vi "InitQueues.vi"(8 "error in (no error)":errorcluster) -> (0 "error out":errorcluster, 3 "Application Data":T1)   [LabVIEW 2019]
uses:
  Typedefs/#cluster_ApplicationData.ctl
  Typedefs/Acquisition Thread/#cluster_AcqQueueData.ctl
  Typedefs/Acquisition Thread/#enum_AcquisitionTask.ctl
  Typedefs/Saving Thread/#cluster_SavingQueueData.ctl
  Typedefs/Saving Thread/#enum_SavingTask.ctl
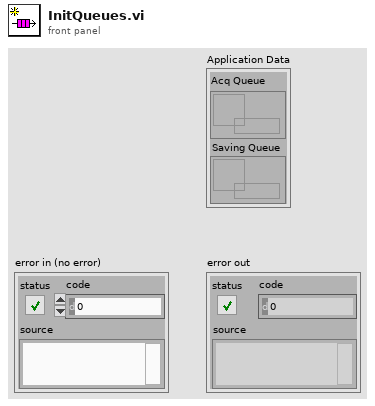
[diagram p1: front panel]
types:
  T1 = typedef "#cluster_ApplicationData.ctl" = cluster{"Acq Queue":refnum<queue>, "Saving Queue":refnum<queue>}
  T2 = typedef "#cluster_SavingQueueData.ctl" = cluster{"Task":T3, "Data":variant}
  T3 = typedef "#enum_SavingTask.ctl" = enum16{"Set directory", "Save", "Stop", "Close"}
  T4 = typedef "#cluster_AcqQueueData.ctl" = cluster{"Task":T5, "Data":variant}
  T5 = typedef "#enum_AcquisitionTask.ctl" = enum16{"Init", "Start", "Finish", "Close"}
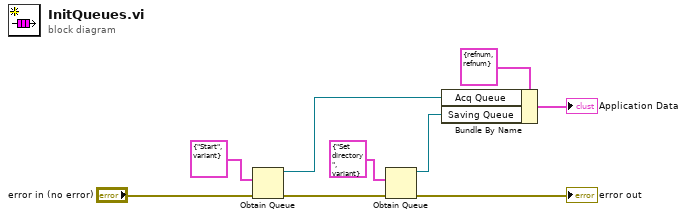
[diagram p0: block diagram]
diagram:
  n1 = Obtain Queue(element data type=T4 {"Task"=enum."Start", "Data"=variant} ("Acq Data"), error in (no error)="error in (no error)") -> (queue out=w5:refnum<queue>, error out=w8:errorcluster)  [unwired: 3 in, 1 out]
  n2 = Obtain Queue(element data type=T2 {"Task"=enum."Set directory", "Data"=variant} ("Saving Data"), error in (no error)=w8) -> (queue out=w4:refnum<queue>, error out=→"error out":errorcluster)  [unwired: 3 in, 1 out]
  n3 = Bundle By Name(cluster=T1 {"Acq Queue"=refnum, "Saving Queue"=refnum} ("App Data"), "Acq Queue"=w5, "Saving Queue"=w4) -> (→"Application Data":T1)
